vi "CANOpen_Get Node Name from ID.vi"(11 "Node ID":u8) -> (3 "Node ID Name":string)   [LabVIEW 2013]
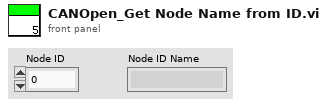
[diagram p1: front panel]
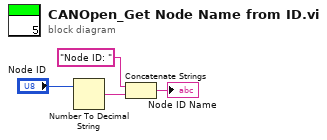
[diagram p0: block diagram]
diagram:
  n1 = Number To Decimal String(number="Node ID") -> (decimal integer string=w4:string)  [unwired: 1 in]
  n2 = Concatenate Strings("Node ID: " ("regular expression"), w4) -> (→"Node ID Name":string)
